vi "Create All Message Queues.vi"(8 "error in (no error)":T1 caption="Fehler (Eingang, kein Fehler)") -> (0 "error out":T1 caption="Fehler (Ausgang)", 3 "Nachrichten-Queues (Ausgang)":T2)   [LabVIEW 2014, in "MyQH Message Queue.lvlib"]
doc: "Dieses VI erstellt und initialisiert alle Nachrichten-Queues Ihrer Anwendung. Klicken Sie zum Hinzufügen von Nachrichten-Queues mit der rechten Maustaste auf die Konstante \"Nachrichten-Queues\" und wählen Sie \"Typdefinition öffnen\". Fügen Sie die neue(n) Queue(s) der Typdefinition hinzu und initialisieren Sie sie in diesem VI."
uses:
  MyQH Message Queue.lvlib
  All Message Queues.ctl
  Message Cluster.ctl
  Enqueue Message (Single).vi
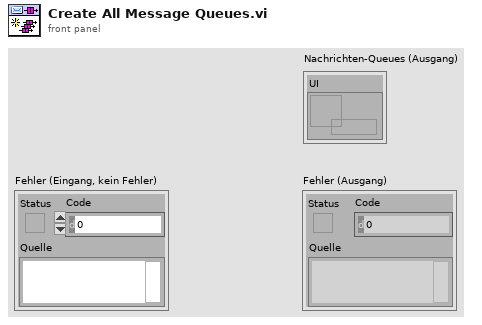
[diagram p1: front panel]
types:
  T1 = cluster{"Status":bool, "Code":i32, "Quelle":string}
  T2 = typedef "MyQH Message Queue.lvlib/All Message Queues.ctl" = cluster{"UI":refnum<queue>}
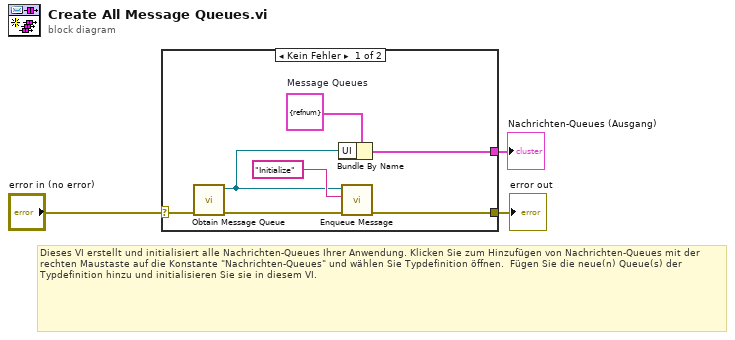
[diagram p0: block diagram]
diagram:
  # "Dieses VI erstellt und initialisiert alle Nachrichten-Queues Ihrer Anwendung. Klicken Sie zum Hinzufügen von Nachrichten-Queues mit der rechten Maustaste auf die Konstante \"Nachrichten-Queues\" und wählen Sie Typdefinition öffnen.  Fügen Sie die neue(n) Queue(s) der Typdefinition hinzu und initialisieren Sie sie in diesem VI."
  n1 = case shown="Kein Fehler" "error in (no error)" {
    selector: "error in (no error)" -> [w7 w11]
    tunnel: [w10 w11] -> w3
    tunnel: [w8 _] -> w2
    frame No Error {
      w9 = T2 {"UI"=refnum}  # Message Queues
      n2 = call "Obtain Message Queue.vi"("error in (no error)"=w7) -> ("error out"=w6:T1, "Nachrichten-Queue"=w4:refnum<queue>)  [unwired: 9 in]
      n3 = Bundle By Name(cluster=w9, "UI"=w4) -> (w8:T2)
      n4 = call-poly "Enqueue Message.vi"("error in (no error)"=w6, "Nachricht"="Initialize" ("Message"), "Nachrichten-Queue"=w4) -> ("error out"=w10:T1)  [unwired: 7 in, 1 out]
    }
    frame Error {
    }
  }
  "Nachrichten-Queues (Ausgang)" <- w2
  "error out" <- w3
